vi "Comments.Create Lockin AO Description.vi"(7 "error in (no error)":errorcluster, 10 "Control Experiment":refnum<class "Control Experiment.lvclass">) -> (0 "error out":errorcluster, 2 "AO Section":string, 3 "Control Experiment out":refnum<class "Control Experiment.lvclass">)   [LabVIEW 2016, in "Control Experiment.lvclass"]
uses:
  Control Experiment.lvclass
  <userlib>/LevyLab/Lockin-Multichannel/Instrument.Lockin/Instrument.Lockin.lvclass
  <userlib>/LevyLab/PLYM/YAML.lvclass
  C:/Program Files (x86)/National Instruments/LabVIEW 2016/user.lib/LevyLab/Levylab Instruments/SMOs/Instrument/Instrument.lvclass
  C:/Program Files (x86)/National Instruments/LabVIEW 2016/vi.lib/JKI/JKI SMO/SMO/SMO.lvclass
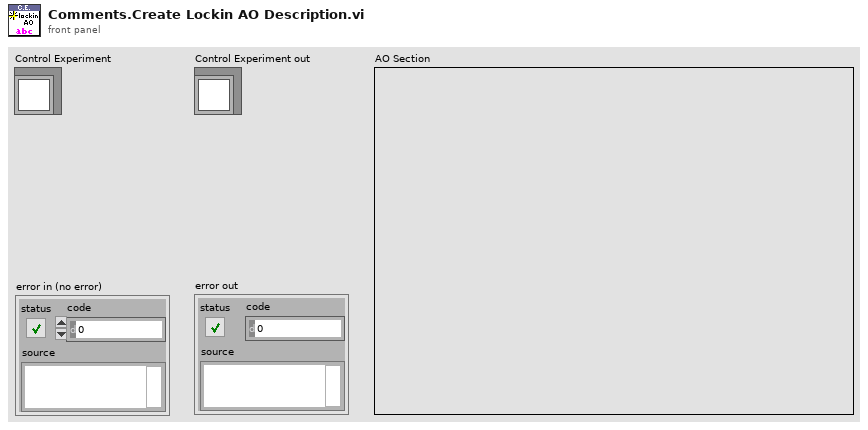
[diagram p1: front panel]
types:
  T1 = typedef "Lockin.DAQ.lvclass/AO-cluster.ctl" = T2[]
  T2 = typedef "Instrument.Lockin.UI.lvclass/AO Channel--Cluster.ctl" = cluster{"Enable?":bool, "Channel":i32, "Amplitude":dbl, "Offset":dbl, "Frequency":dbl, "Phase":dbl, "Function":T3, "Sweeping?":bool}
  T3 = typedef "Lockin.DAQ.lvclass/Function-enum.ctl" = enum16{"Sine", "Triangle", "Square"}
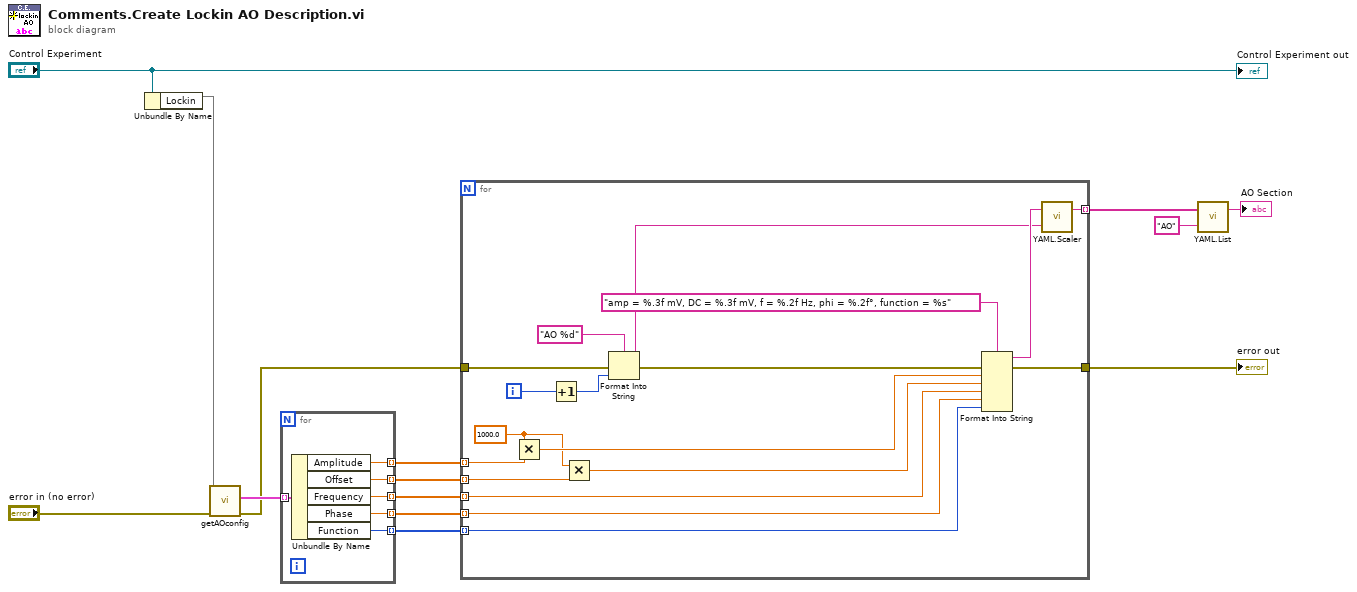
[diagram p0: block diagram]
diagram:
  n1 = Unbundle By Name("Control Experiment") -> ("Lockin"=w2)
  n2 = call <userlib>:"getAOconfig.vi"("error in (no error)"="error in (no error)", "Instrument.Lockin in"=w2) -> ("error out"=w3:errorcluster, "AOconfig"=w4:T1)  [unwired: 7 in, 1 out]
  n3 = for {
    tunnel: [w20] -> w10 mode=indexing
    tunnel: [w19] -> w9 mode=indexing
    tunnel: [w18] -> w8 mode=indexing
    tunnel: [w17] -> w7 mode=indexing
    tunnel: [w16] -> w6 mode=indexing
    tunnel: w4 -> [w15] mode=indexing
    n4 = Unbundle By Name(w15) -> ("Amplitude"=w20:dbl, "Offset"=w19:dbl, "Frequency"=w18:dbl, "Phase"=w17:dbl, "Function"=w16:T3)
  }
  n5 = for {
    tunnel: w10 -> [w30] mode=indexing
    tunnel: w9 -> [w31] mode=indexing
    tunnel: w8 -> [w24] mode=indexing
    tunnel: w7 -> [w23] mode=indexing
    tunnel: w6 -> [w22] mode=indexing
    tunnel: [w26] -> w5 mode=indexing
    tunnel: w3 -> [w38]
    tunnel: [w36] -> w14
    i -> [w35]
    w28 = 1000.0 ("x")
    n6 = Multiply(x=w28, y=w30) -> (x*y=w29:dbl)
    n7 = Increment(x=w35) -> (x+1=w21:i32)
    n8 = Multiply(x=w28, y=w31) -> (x*y=w25:dbl)
    n9 = Format Into String(format string="AO %d", error in=w38, w21) -> (resulting string=w27:string, error out=w37:errorcluster)  [unwired: 1 in]
    n10 = Format Into String(format string="amp = %.3f mV, DC = %.3f mV, f = %.2f Hz, phi = %.2f°, function = %s", error in=w37, w29, w25, w24, w23, w22) -> (resulting string=w32:string, error out=w36:errorcluster)  [unwired: 1 in]
    n11 = call <userlib>:"YAML.Scaler.vi"("Key"=w27, "Scaler"=w32) -> ("Output"=w26:string)  [unwired: 1 in]
  }
  "error out" <- w14
  n12 = call <userlib>:"YAML.List.vi"("Key"="AO" ("string"), "lines"=w5) -> ("Output"=→"AO Section":string)  [unwired: 1 in]
  "Control Experiment out" <- "Control Experiment"
